vi "Addition Example.vi"() -> ()   [LabVIEW 2018]
panel:
  in  "3nd":dbl
  in  "1st Number":dbl
  out "output":dbl
  in  "input 2":dbl
  in  "input 1":dbl
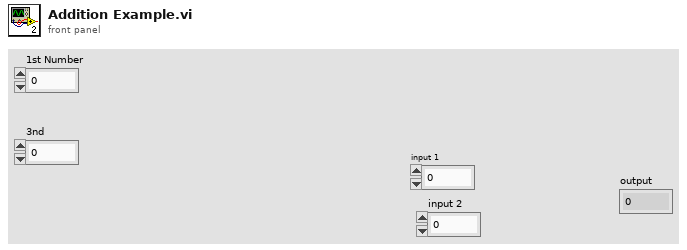
[diagram p1: front panel]
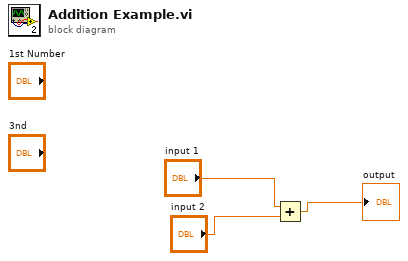
[diagram p0: block diagram]
diagram:
  n1 = Add(x="input 1", y="input 2") -> (x+y=→"output":dbl)
